vi "createhtml.vi"() -> ()   [LabVIEW 2010]
uses:
  <vilib>/Analysis/NI_AALBase.lvlib
panel:
  in  "停止":bool
  out "波形图":dbl[](graph)
  in  "幅值":dbl(slide)=1.0 scale=0.0..10.0
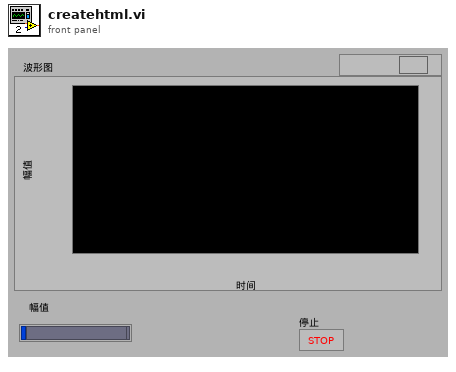
[diagram p1: front panel]
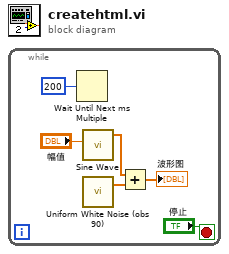
[diagram p0: block diagram]
diagram:
  n1 = while {
    stop <- "停止" stop-if-true
    n2 = Wait Until Next ms Multiple(millisecond multiple=u32 200) -> ()  [unwired: 1 out]
    n3 = call <vilib>:"Sine Wave.vi"("amplitude"="幅值") -> ("sine wave"=w5:dbl[])  [unwired: 4 in, 2 out]
    n4 = call <vilib>:"Uniform White Noise (obs 90).vi"() -> ("uniform white noise"=w2:dbl[])  [unwired: 3 in, 1 out]
    n5 = Add(x=w5, y=w2) -> (x+y=→"波形图":dbl[])
  }
